vi "Stato strumenti.vi"(8 "error in (no error)":errorcluster, 11 "Indice":i32) -> ()   [LabVIEW 2019]
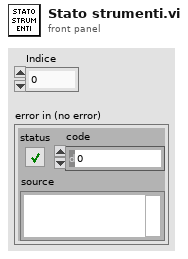
[diagram p1: front panel]
types:
  T1 = cluster{"Message":string, "Message Data":variant}
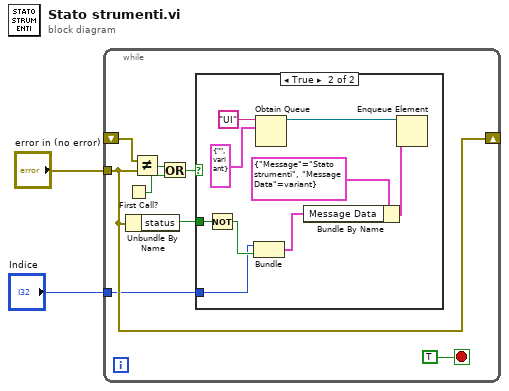
[diagram p0: block diagram]
diagram:
  n1 = while {
    shift-right: [w5] -> _
    shift-left: _ -> [w9]
    tunnel: "error in (no error)" -> [w5]
    tunnel: "Indice" -> [w3]
    stop <- TRUE stop-if-true
    n2 = First Call?() -> (First Call?: T/F=w6:bool)
    n3 = Unbundle By Name(w5) -> ("status"=w4:bool)
    n4 = Not Equal?(x=w9, y=w5) -> (x != y?=w8:bool)
    n5 = Or(x=w8, y=w6) -> (x .or. y?=w7:bool)
    n6 = case shown="True" w7 {
      tunnel: w4 -> [_ w14]
      tunnel: w3 -> [_ w12]
      frame False {
      }
      frame True {
        n7 = Not(x=w14) -> (.not. x?=w13:bool)
        n8 = Bundle("Indice"=w12, w13) -> (w11:cluster{"Indice":i32, bool})  [unwired: 1 in]
        n9 = Obtain Queue(name (unnamed)="UI", element data type=T1 {"Message"="", "Message Data"=variant} ("Message Cluster")) -> (queue out=w17:refnum<queue>)  [unwired: 3 in, 2 out]
        n10 = Bundle By Name(cluster=T1 {"Message"="Stato strumenti", "Message Data"=variant} ("Message Cluster"), "Message Data"=w11) -> (w15:T1)
        n11 = Enqueue Element(queue=w17, element=w15) -> ()  [unwired: 2 in, 3 out]
      }
    }
  }
